vi "401_Decending.vi"(11 "Data_Table":string[][](array[string])) -> (3 "Array":string[][](array[string]))   [LabVIEW 2015]
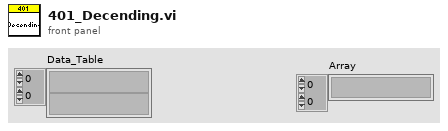
[diagram p1: front panel]
types:
  T1 = cluster{string, string, string, string, string, string, string}[]
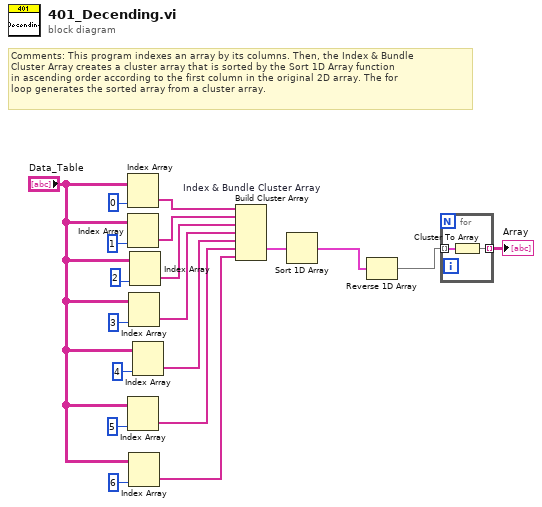
[diagram p0: block diagram]
diagram:
  # "Comments: This program indexes an array by its columns. Then, the Index & Bundle\nCluster Array creates a cluster array that is sorted by the Sort 1D Array function\nin ascending order according to the first column in the original 2D array. The for\nloop generates the sorted array from a cluster array."
  n1 = Index Array(array="Data_Table", index (col)=0) -> (element=w19:string[])  [unwired: 1 in]
  n2 = Index Array(array="Data_Table", index (col)=1) -> (element=w18:string[])  [unwired: 1 in]
  n3 = Index Array(array="Data_Table", index (col)=5) -> (element=w4:string[])  [unwired: 1 in]
  n4 = Index Array(array="Data_Table", index (col)=3) -> (element=w8:string[])  [unwired: 1 in]
  n5 = Index Array(array="Data_Table", index (col)=6) -> (element=w2:string[])  [unwired: 1 in]
  n6 = Index Array(array="Data_Table", index (col)=2) -> (element=w9:string[])  [unwired: 1 in]
  n7 = Index Array(array="Data_Table", index (col)=4) -> (element=w6:string[])  [unwired: 1 in]
  n8 = Build Cluster Array "Index & Bundle Cluster Array"(w19, w18, w9, w8, w6, w4, w2) -> (w17:T1)
  n9 = Sort 1D Array(array=w17) -> (sorted array=w13:T1)
  n10 = Reverse 1D Array(array=w13) -> (reversed array=w12:T1)
  n11 = for {
    tunnel: w12 -> [w21] mode=indexing
    tunnel: [w20] -> w14 mode=indexing
    n12 = Cluster To Array(cluster=w21) -> (array=w20:string[])
  }
  "Array" <- w14
